vi "ApplyModifiers.vi"(8 "error in (no error)":errorcluster, 10 "modifiers":T2[](array[typedef]), 11 "node in":refnum<k20>) -> (0 "error out":errorcluster, 2 "properties":T1[](array[typedef]), 3 "node out":refnum<k20>)   [LabVIEW 2015, in "VeriStandTestUtilities.lvlib"]
uses:
  VeriStandTestUtilities.lvlib
  ConfigurationItem.ctl
  ConfigurationItemType.ctl
  OverrideItem.ctl
  PropertyItem.ctl
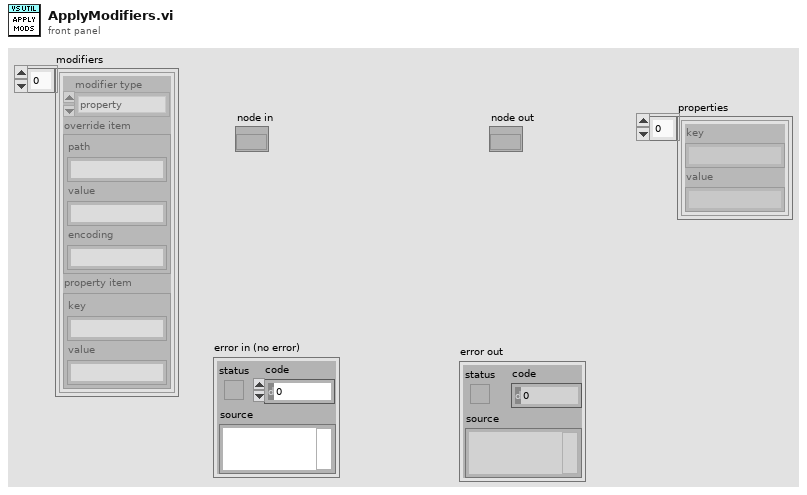
[diagram p1: front panel]
types:
  T1 = typedef "VeriStandTestUtilities.lvlib/PropertyItem.ctl" = cluster{"key":string, "value":string}
  T2 = typedef "VeriStandTestUtilities.lvlib/ConfigurationItem.ctl" = cluster{"modifier type":T3, "override item":T4, "property item":cluster{"key":string, "value":string}}
  T3 = typedef "VeriStandTestUtilities.lvlib/ConfigurationItemType.ctl" = enum16{"property", "override"}
  T4 = typedef "VeriStandTestUtilities.lvlib/OverrideItem.ctl" = cluster{"path":string, "value":string, "encoding":string}
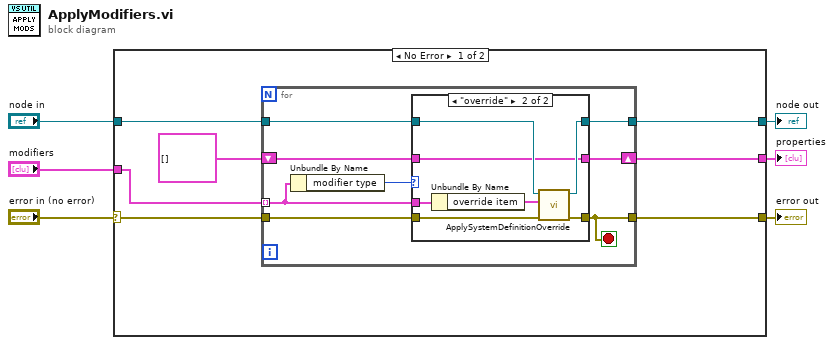
[diagram p0: block diagram]
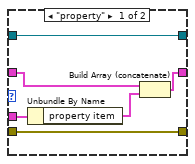
[diagram p2: hidden frame]
diagram:
  n1 = case shown="No Error" "error in (no error)" {
    selector: "error in (no error)" -> [w12 w36]
    tunnel: [w11 w36] -> w6
    tunnel: "modifiers" -> [w13 _]
    tunnel: "node in" -> [w10 w35]
    tunnel: [w9 w35] -> w2
    tunnel: [w7 _] -> w1
    frame No Error {
      n2 = for {
        tunnel: w13 -> [w17] mode=indexing
        tunnel: w12 -> [w20]
        tunnel: [w14] -> w11
        tunnel: w10 -> [w19]
        tunnel: [w18] -> w9
        shift-right: [w15] -> w7
        shift-left: T1[] [] -> [w16]
        stop <- w14 stop-if-true
        n3 = Unbundle By Name(w17) -> ("modifier type"=w21:T3)
        n4 = case shown="\"override\"" w21 {
          tunnel: w20 -> [w27 w34]
          tunnel: [w27 w33] -> w14
          tunnel: w19 -> [w26 w32]
          tunnel: [w26 w31] -> w18
          tunnel: w17 -> [w25 w30]
          tunnel: w16 -> [w23 w28]
          tunnel: [w22 w28] -> w15
          frame "property" {
            n5 = Unbundle By Name(w25) -> ("property item"=w24:cluster{"key":string, "value":string})
            n6 = Build Array (concatenate)(w23, w24) -> (w22:T1[])
          }
          frame "override" {
            n7 = Unbundle By Name(w30) -> ("override item"=w29:T4)
            n8 = call "ApplySystemDefinitionOverride.vi"("error in (no error)"=w34, "override item"=w29, "node in"=w32) -> ("error out"=w33:errorcluster, "node out"=w31:refnum<k20>)  [unwired: 7 in]
          }
        }
      }
    }
    frame Error {
    }
  }
  "error out" <- w6
  "node out" <- w2
  "properties" <- w1
